vi "SampleToHexString.vi"(11 "Sample":T1) -> (3 "StringOut":string)   [LabVIEW 2016]
doc: "Convert measurement data to string."
uses:
  FallSensor/Sample.ctl
  FallSensor/Reading.ctl
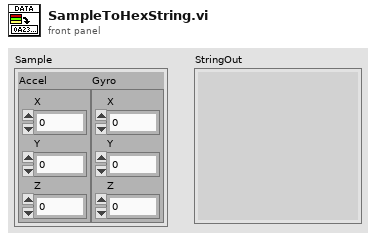
[diagram p1: front panel]
types:
  T1 = typedef "Sample.ctl" = cluster{"Accel":T2, "Gyro":T2}
  T2 = typedef "Reading.ctl" = cluster{"X":i16, "Y":i16, "Z":i16}
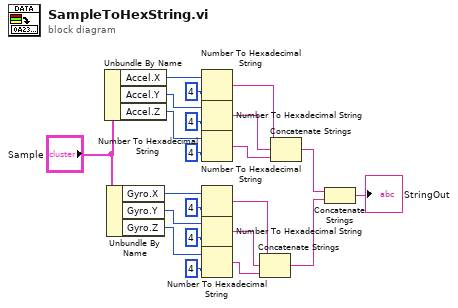
[diagram p0: block diagram]
diagram:
  n1 = Unbundle By Name("Sample") -> ("Accel.X"=w21:i16, "Accel.Y"=w17:i16, "Accel.Z"=w16:i16)
  n2 = Unbundle By Name("Sample") -> ("Gyro.X"=w10:i16, "Gyro.Y"=w14:i16, "Gyro.Z"=w15:i16)
  n3 = Number To Hexadecimal String(1:i16 4 ("width (-)"), 2:w21) -> (0:w9:string)
  n4 = Number To Hexadecimal String(1:i16 4 ("width (-)"), 2:w17) -> (0:w8:string)
  n5 = Number To Hexadecimal String(1:i16 4 ("width (-)"), 2:w16) -> (0:w7:string)
  n6 = Number To Hexadecimal String(1:i16 4 ("width (-)"), 2:w10) -> (0:w4:string)
  n7 = Number To Hexadecimal String(1:i16 4 ("width (-)"), 2:w14) -> (0:w5:string)
  n8 = Number To Hexadecimal String(1:i16 4 ("width (-)"), 2:w15) -> (0:w6:string)
  n9 = Concatenate Strings(w4, w5, w6) -> (w3:string)
  n10 = Concatenate Strings(w9, w8, w7) -> (w2:string)
  n11 = Concatenate Strings(w2, w3) -> (→"StringOut":string)
